vi "Periodic Tasks.vi"(8 "error in":errorcluster) -> ()   [LabVIEW 2017]
doc: "This VI runs in parallel to other tasks. It can contain as many user-defined periodic loops as you need. These can carry out PID or other sorts of timed response."
uses:
  <vilib>/Rock Robotics/WPI/DriverStation/WPI_DriverStationRobotMode2.ctl
  Robot Global Data.vi
  <vilib>/Rock Robotics/Network Tables/NT Write Boolean.vi
  Public/Documents/Cross The Road Electronics/Phoenix-LabVIEW/Motor Controller/Get/CTRE_Phoenix_MotorController_GetPulseWidthAll.vi
  <vilib>/Rock Robotics/Network Tables/NT Write Number.vi
  <vilib>/Rock Robotics/Network Tables/NT Read Boolean Array.vi
  <vilib>/Rock Robotics/Network Tables/NT Write Numeric Array.vi
  <vilib>/Utility/file.llb/Write Delimited Spreadsheet (DBL).vi
  <vilib>/Utility/file.llb/Read Delimited Spreadsheet (DBL).vi
  <vilib>/Rock Robotics/Network Tables/NT Read String.vi
  <vilib>/Rock Robotics/Network Tables/NT Write String.vi
  <vilib>/Rock Robotics/Network Tables/NT Read Numeric Array.vi
  <vilib>/Rock Robotics/Network Tables/NT Read Boolean.vi
  <vilib>/Rock Robotics/Network Tables/NT Read String Array.vi
  <vilib>/Rock Robotics/Network Tables/NT Write String Array.vi
panel:
  in  "Zero Gyro":bool
  in  "Enable Graphs":bool
  out "FL Drive":dbl(graph)
  out "FR Drive":dbl(graph)
  out "BL Drive 2":dbl(graph)
  out "BR Drive 2":dbl(graph)
  out "FL Spin 2":dbl(graph)
  out "BL Spin 3":dbl(graph)
  out "FR Spin 2":dbl(graph)
  out "BR Spin 3":dbl(graph)
  in  "Reset Lift at Start Config":bool
  in  "Disable DB Config Writing":bool
  in  "Save Zeros to File":bool
  in  "Read Zeros from File":bool
  in  "Zero Drive":bool
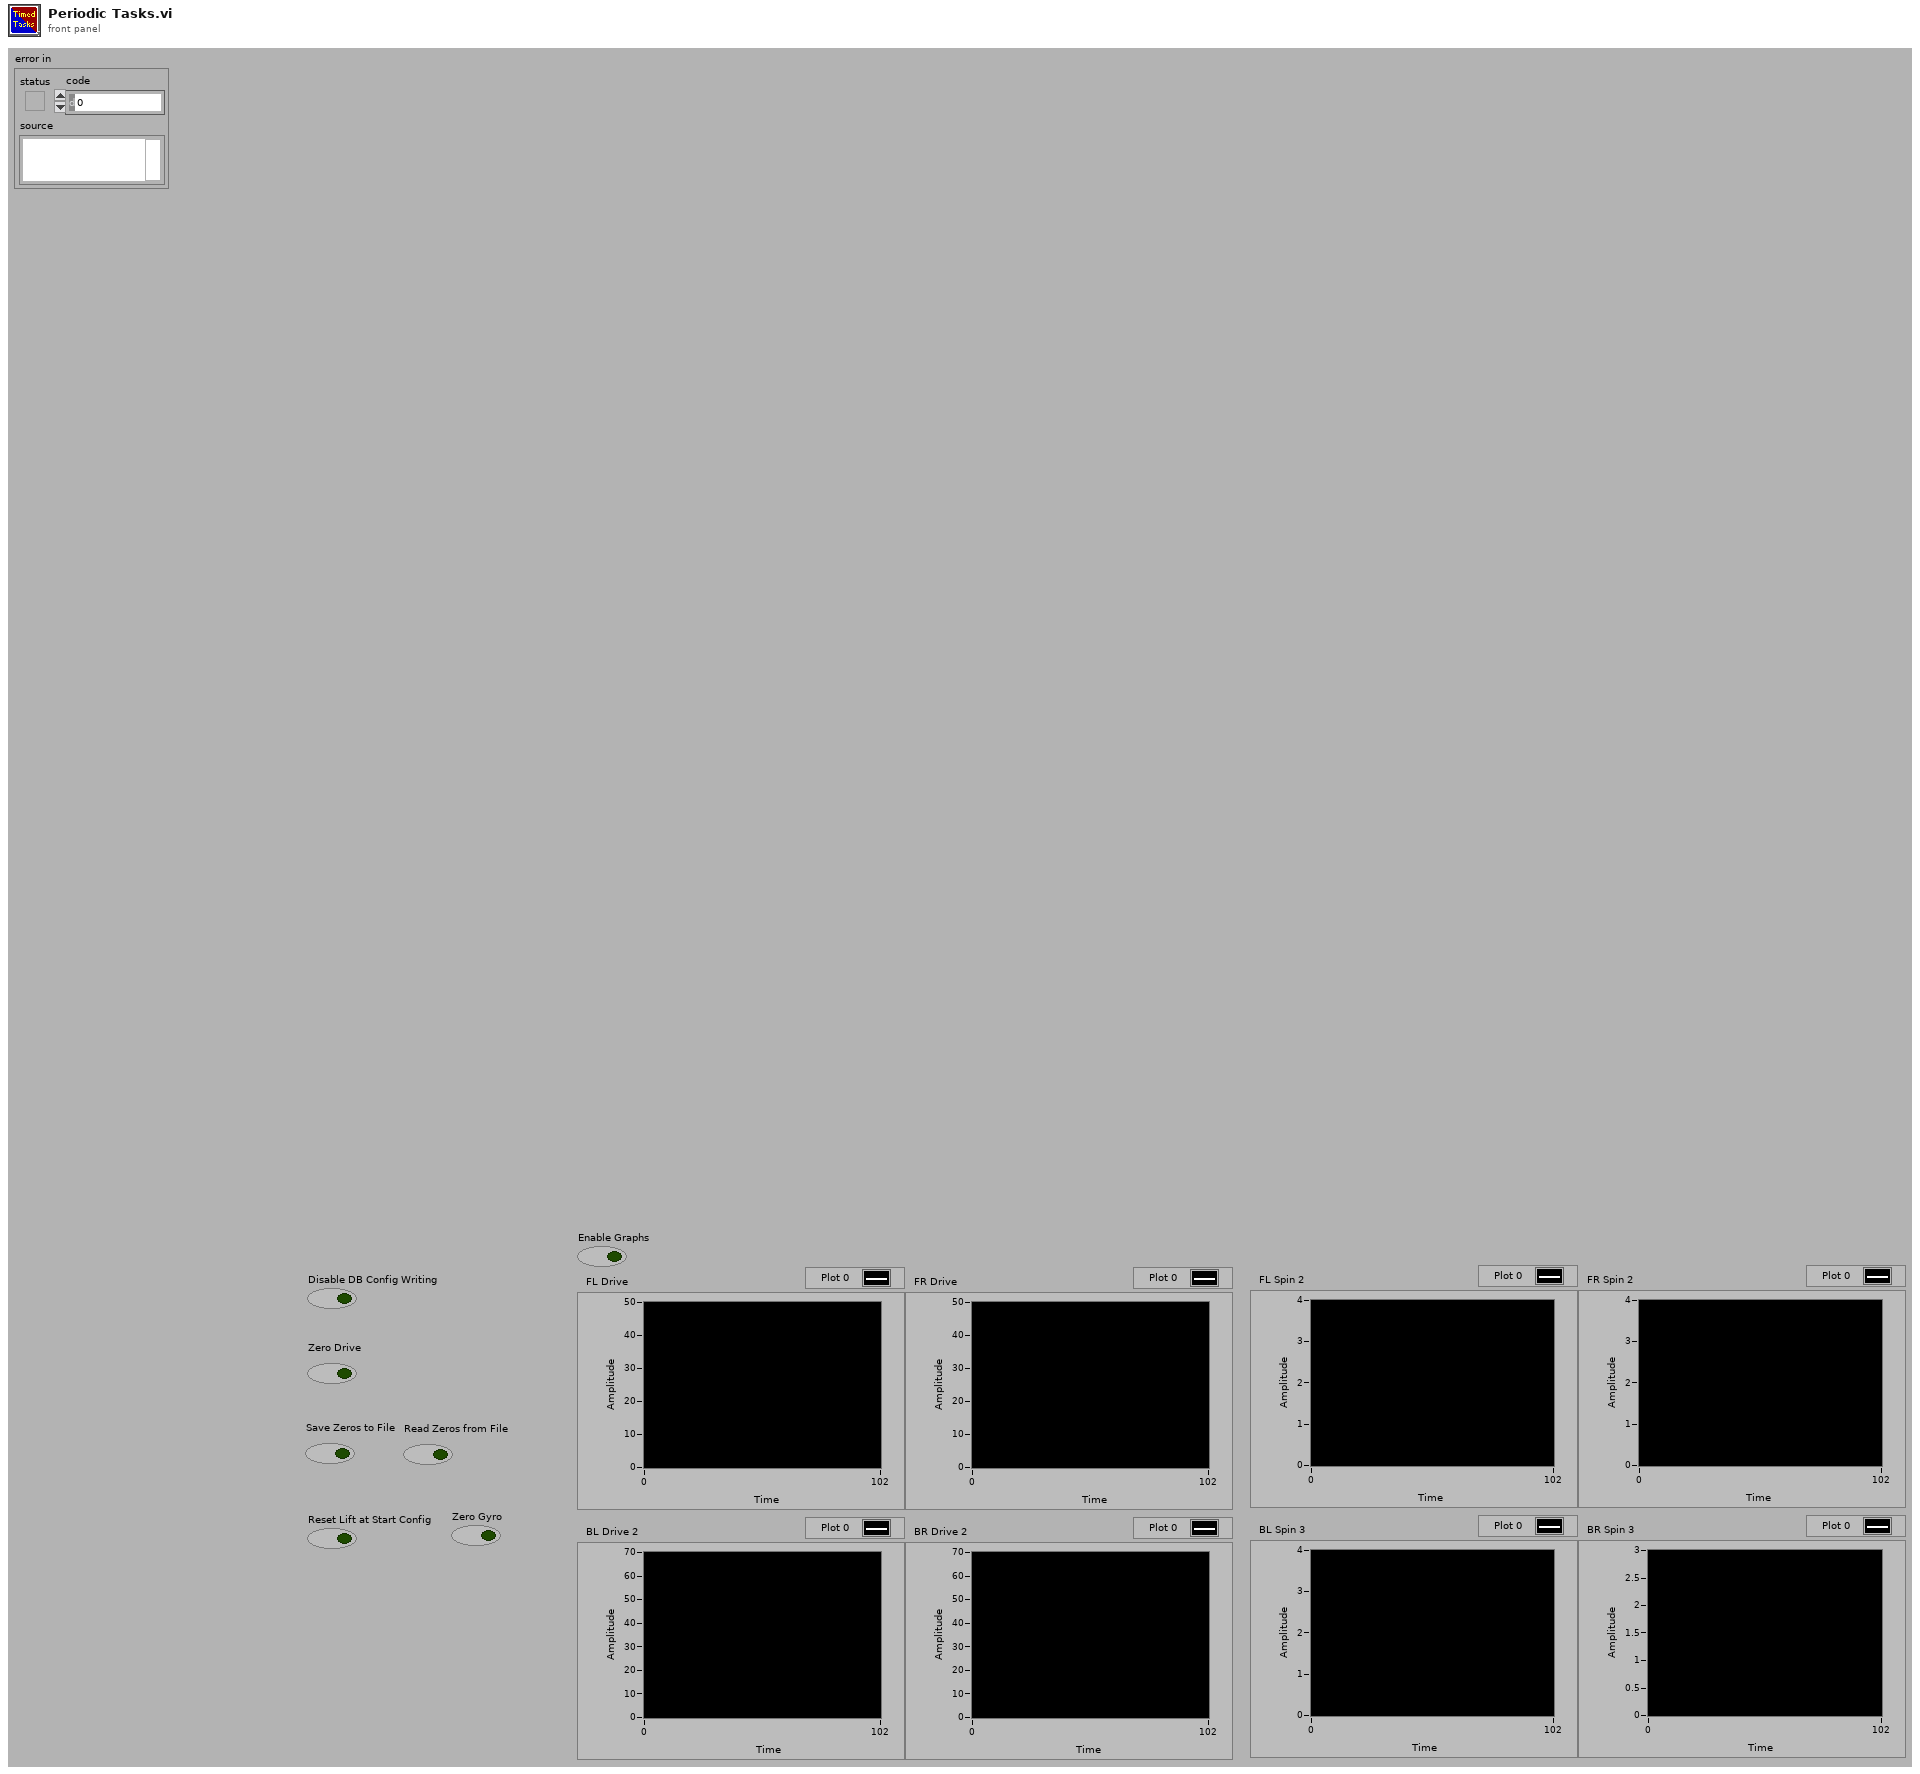
[diagram p1: front panel]
types:
  T1 = typedef "WPI_DriverStationRobotMode2.ctl" = enum16{"Autonomous Disabled", "Autonomous Enabled", "Teleop Disabled", "Teleop Enabled", "Disconnected", "Finish", "Test Disabled", "Test Enabled", "Emergency Stopped"}
  T2 = typedef "WPI_MotorControlDeviceRef.ctl" = cluster{"DeviceStatus":errorcluster, "Type":T3, "PWM":cluster{"PWM Channel":T4, "DeadBand":T5}, "CAN":cluster{"Device Number":u8, "SetOutput VI Ref":variant, "GetOutput VI Ref":variant, "Enable VI Ref":variant, "Disable VI Ref":variant, "Data":variant}, "Invert":bool, "DIO PWM":cluster{"PWM \"Enable\" Channel":T4, "DIOChannel":T6, "PWM Rate":dbl}}
  T3 = typedef "WPI_MotorControlType.ctl" = enum16{"PWM", "CAN", "DIO PWM"}
  T4 = typedef "FPGA_DIOPWMChannel.ctl" = enum8{"PWM 0", "PWM 1", "PWM 2", "PWM 3", "PWM 4", "PWM 5", "PWM 6", "PWM 7", "PWM 8", "PWM 9", "PWM MXP 0", "PWM MXP 1", "PWM MXP 2", "PWM MXP 3", "PWM MXP 4", "PWM MXP 5", "PWM MXP 6", "PWM MXP 7", "PWM MXP 8", "PWM MXP 9", "Invalid"}
  T5 = typedef "WPI_PWMDeadband.ctl" = cluster{"Name":string, "maxPositivePwm":i32, "minPositivePwm":i32, "centerPwm":i32, "maxNegativePwm":i32, "minNegativePwm":i32, "angularRange":u16}
  T6 = typedef "FPGA_DIOChannel.ctl" = enum8{"DIO 0", "DIO 1", "DIO 2", "DIO 3", "DIO 4", "DIO 5", "DIO 6", "DIO 7", "DIO 8", "DIO 9", "DIO MXP 0", "DIO MXP 1", "DIO MXP 2", "DIO MXP 3", "DIO MXP 4", "DIO MXP 5", "DIO MXP 6", "DIO MXP 7", "DIO MXP 8", "DIO MXP 9", "DIO MXP 10", "DIO MXP 11", "DIO MXP 12", "DIO MXP 13", "DIO MXP 14", "DIO MXP 15", "SPI Port CS1", "SPI Port CS2", "SPI Port CS3", "SPI Port MISO", "SPI Port MOSI", "Invalid"}
  T7 = typedef "WPI_SwitchDevRef.ctl" = cluster{"DevStatus":errorcluster, "DIO Channel":T6, "CntIndex":T8, "Normally Closed":bool}
  T8 = typedef "FPGA_CounterCtrSystemIndex.ctl" = enum8{"Ctr 0", "Ctr 1", "Ctr 2", "Ctr 3", "Ctr 4", "Ctr 5", "Ctr 6", "Ctr 7", "Invalid"}
  T9 = cluster{"Yaw":dbl, "Roll":dbl, "Pitch":dbl, "Heading":dbl, "Fused Heading":dbl}
  T10 = typedef "WPI_EncoderDevRef.ctl" = cluster{"DevStatus":errorcluster, "EncoderIndex":T11, "CounterIndex":T8, "DistancePerCount":dbl, "Decoding Type":T12}
  T11 = typedef "FPGA_EncoderIdx.ctl" = enum8{"Enc 0", "Enc 1", "Enc 2", "Enc 3", "Enc 4", "Enc 5", "Enc 6", "Enc 7", "Invalid"}
  T12 = typedef "WPI_EncoderType.ctl" = enum16{"1x", "2x", "4x"}
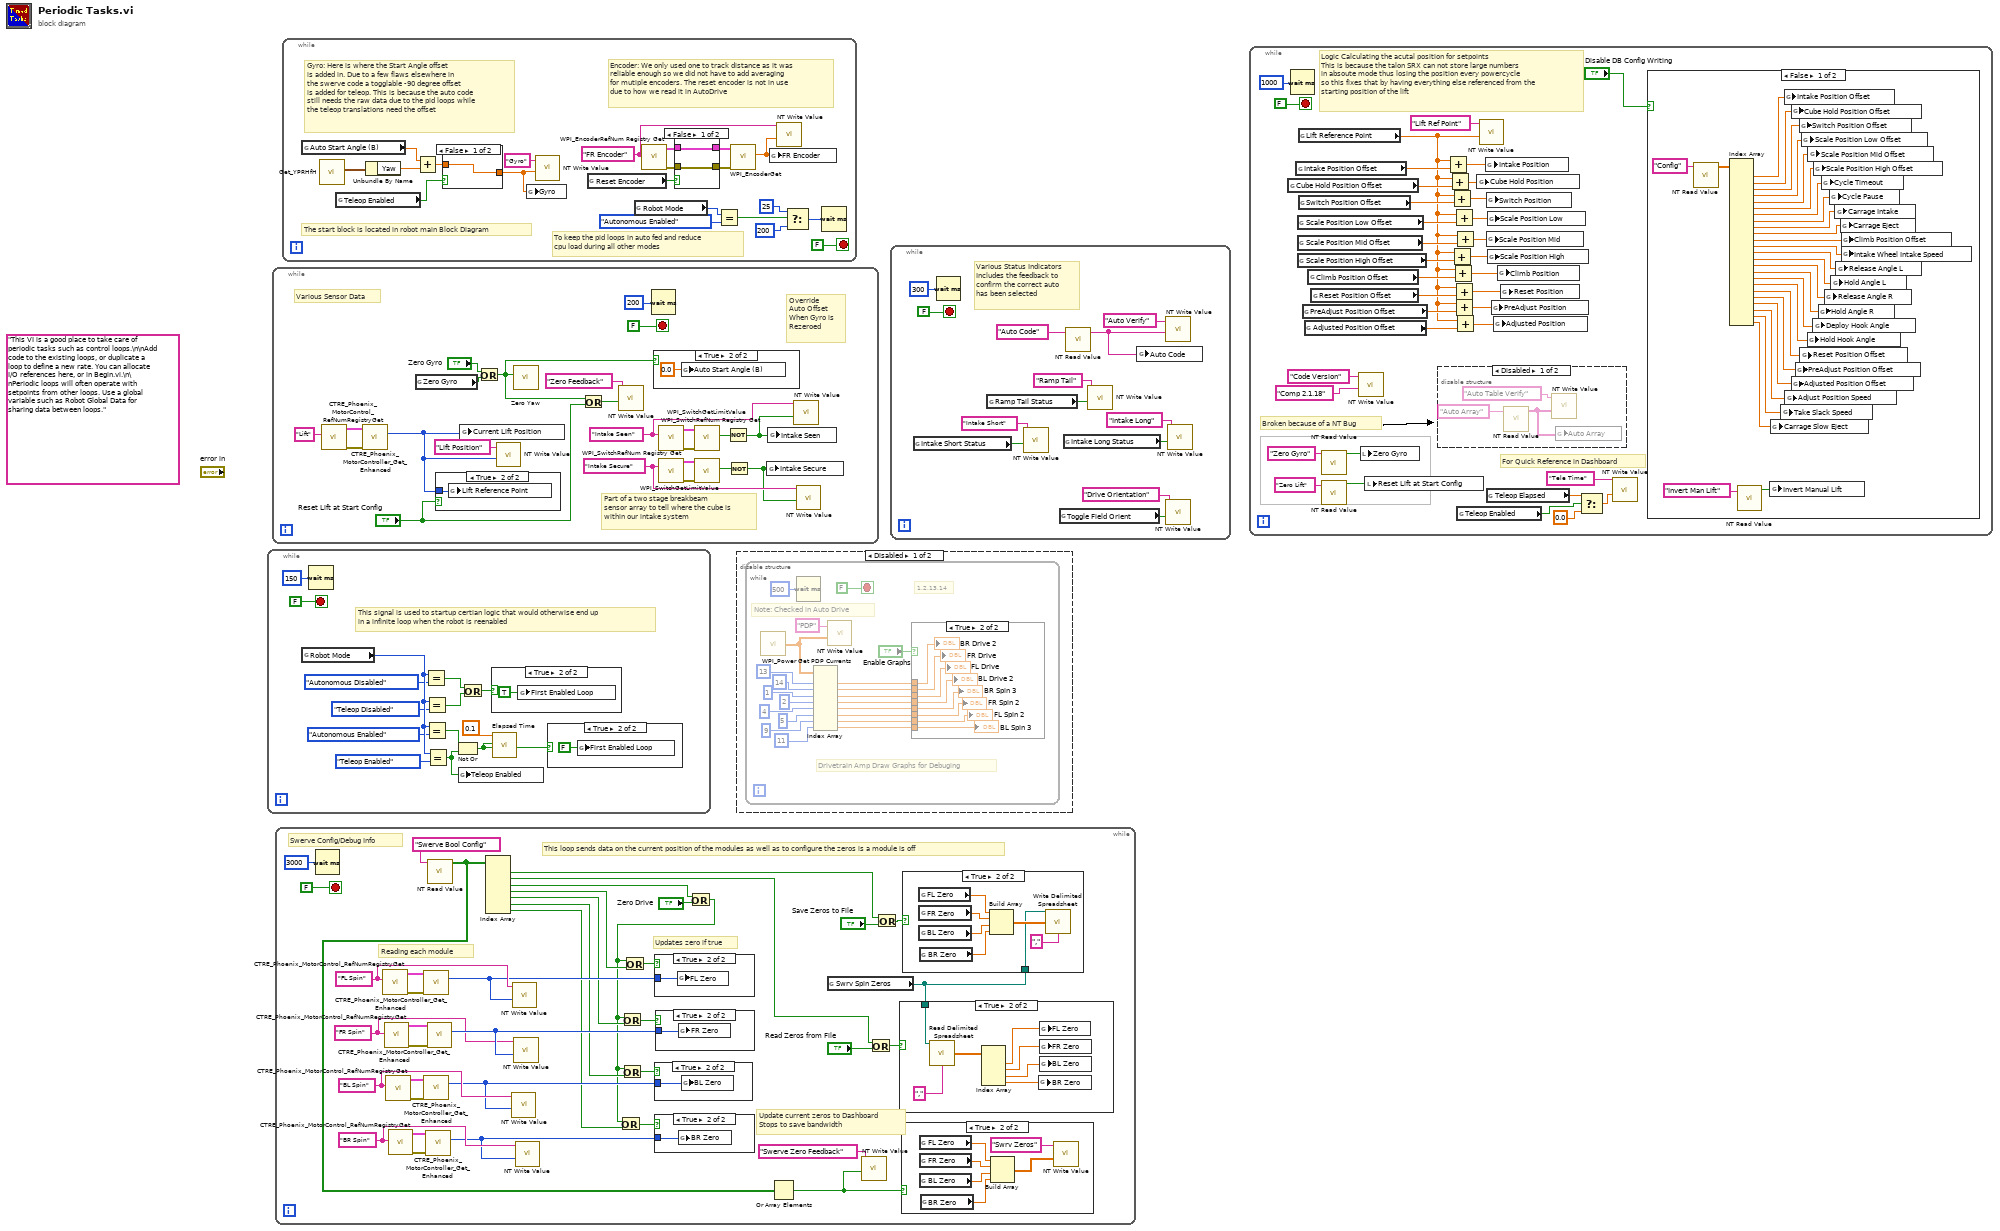
[diagram p0: block diagram]
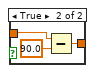
[diagram p2: hidden frame]
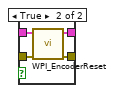
[diagram p3: hidden frame]
diagram:
  (unwired) "This VI is a good place to take care of periodic tasks such as control loops.\n\nAdd code to the existing loops, or duplicate a loop to define a new rate. You can allocate I/O references here, or in Begin.vi.\n\nPeriodic loops will often operate with setpoints from other loops. Use a global variable such as Robot Global Data for sharing data between loops."
  n1 = while {
    stop <- FALSE stop-if-true
    # "This signal is used to startup certian logic that would otherwise end up \nin a infinite loop when the robot is reenabled"
    n2 = global read "Robot Global Data.vi" "Robot Mode"() -> (w7:T1)
    n3 = Wait (ms)(milliseconds to wait=u32 150) -> ()  [unwired: 1 out]
    n4 = Equal?(x=w7, y=WPI_DriverStationRobotMode2."Autonomous Disabled") -> (x = y?=w8:bool)
    n5 = Equal?(x=w7, y=WPI_DriverStationRobotMode2."Teleop Disabled") -> (x = y?=w9:bool)
    n6 = Equal?(x=w7, y=WPI_DriverStationRobotMode2."Autonomous Enabled") -> (x = y?=w10:bool)
    n7 = Equal?(x=w7, y=WPI_DriverStationRobotMode2."Teleop Enabled") -> (x = y?=w1:bool)
    n8 = Not Or(1:w1, 2:w10) -> (0:w12:bool)
    n9 = global write "Robot Global Data.vi" "Teleop Enabled"(w1) -> ()
    n10 = Or(x=w8, y=w9) -> (x .or. y?=w11:bool)
    n11 = case shown="True" w11 {
      frame False {
      }
      frame True {
        n12 = global write "Robot Global Data.vi" "First Enabled Loop"(TRUE ("First Enabled Loop")) -> ()
      }
    }
    n13 = call "Elapsed Time"("Time Target (s)"=0.1, "Reset"=w12, "Auto Reset"=w12) -> ("Time has Elapsed"=w13:bool)  [unwired: 9 in, 7 out]
    n14 = case shown="True" w13 {
      frame False {
      }
      frame True {
        n15 = global write "Robot Global Data.vi" "First Enabled Loop"(FALSE ("First Enabled Loop")) -> ()
      }
    }
  }
  n16 = while {
    stop <- FALSE stop-if-true
    w32 = "Intake Secure" ("refnum name")
    w31 = "Intake Seen" ("refnum name")
    # "Part of a two stage breakbeam\nsensor array to tell where the cube is\nwithin our intake system"
    # "Override\nAuto Offset\nWhen Gyro is\nRezeroed"
    # "Various Sensor Data"
    n17 = call "CTRE_Phoenix_MotorControl_RefNumRegistryGet.vi"("refnum name"="Lift") -> ("error out"=w28:errorcluster, "PhoenixMotorControlDevRef"=w29:T2)  [unwired: 9 in]
    n18 = call-poly "CTRE_Phoenix_MotorController_Get_Enhanced.vi"("PhoenixMotorControlDevRef"=w29, "error in"=w28) -> ("Pulse Width Position"=w23:i32)  [unwired: 8 in, 5 out]
    n19 = global read "Robot Global Data.vi" "Zero Gyro"() -> (w20:bool)
    n20 = case shown="True" "Reset Lift at Start Config" {
      tunnel: w23 -> [_ w42]
      frame False {
      }
      frame True {
        n21 = global write "Robot Global Data.vi" "Lift Reference Point"(w42) -> ()
      }
    }
    n22 = global write "Robot Global Data.vi" "Current Lift Position"(w23) -> ()
    n23 = Or(x="Zero Gyro", y=w20) -> (x .or. y?=w18:bool)
    n24 = call-poly <vilib>:"NT Write Value.vi"("Numeric"=w23, "Name"="Lift Position") -> ()  [unwired: 9 in, 1 out]
    n25 = call <vilib>:"Zero Yaw.vi"("Zero"=w18) -> ()  [unwired: 11 in]
    n26 = Or(x=w18, y="Reset Lift at Start Config") -> (x .or. y?=w21:bool)
    n27 = call-poly <vilib>:"NT Write Value.vi"("Boolean"=w21, "Name"="Zero Feedback") -> ()  [unwired: 9 in, 1 out]
    n28 = Wait (ms)(milliseconds to wait=u32 200) -> ()  [unwired: 1 out]
    n29 = case shown="True" w18 {
      frame False {
      }
      frame True {
        n30 = global write "Robot Global Data.vi" "Auto Start Angle (B)"(0.0 ("Auto Start Angle (B)")) -> ()
      }
    }
    n31 = call <vilib>:"WPI_SwitchRefNum Registry Get.vi"("refnum name"=w31) -> ("error out"=w37:errorcluster, "SwitchDevRef"=w36:T7)  [unwired: 9 in]
    n32 = call <vilib>:"WPI_SwitchRefNum Registry Get.vi"("refnum name"=w32) -> ("error out"=w35:errorcluster, "SwitchDevRef"=w34:T7)  [unwired: 9 in]
    n33 = call <vilib>:"WPI_SwitchGetLimitValue.vi"("error in (no error)"=w37, "SwitchDevRef"=w36) -> ("Switch Pressed"=w38:bool)  [unwired: 7 in, 2 out]
    n34 = call <vilib>:"WPI_SwitchGetLimitValue.vi"("error in (no error)"=w35, "SwitchDevRef"=w34) -> ("Switch Pressed"=w33:bool)  [unwired: 7 in, 2 out]
    n35 = Not(x=w38) -> (.not. x?=w26:bool)
    n36 = Not(x=w33) -> (.not. x?=w25:bool)
    n37 = global write "Robot Global Data.vi" "Intake Secure"(w25) -> ()
    n38 = global write "Robot Global Data.vi" "Intake Seen"(w26) -> ()
    n39 = call-poly <vilib>:"NT Write Value.vi"("Boolean"=w26, "Name"=w31) -> ()  [unwired: 9 in, 1 out]
    n40 = call-poly <vilib>:"NT Write Value.vi"("Boolean"=w25, "Name"=w32) -> ()  [unwired: 9 in, 1 out]
  }
  n41 = while {
    stop <- FALSE stop-if-true
    w65 = "BR Spin" ("refnum name")
    w67 = "BL Spin" ("refnum name")
    w68 = "FR Spin" ("refnum name")
    w71 = "FL Spin" ("refnum name")
    # "Reading each module"
    # "Updates zero if true"
    # "This loop sends data on the current position of the modules as well as to configure the zeros is a module is off"
    # "Update current zeros to Dashboard\nStops to save bandwidth"
    # "Swerve Config/Debug Info"
    n42 = Wait (ms)(milliseconds to wait=u32 3000) -> ()  [unwired: 1 out]
    n43 = call "CTRE_Phoenix_MotorControl_RefNumRegistryGet.vi"("refnum name"=w71) -> ("error out"=w73:errorcluster, "PhoenixMotorControlDevRef"=w72:T2)  [unwired: 9 in]
    n44 = call "CTRE_Phoenix_MotorControl_RefNumRegistryGet.vi"("refnum name"=w68) -> ("error out"=w75:errorcluster, "PhoenixMotorControlDevRef"=w74:T2)  [unwired: 9 in]
    n45 = call "CTRE_Phoenix_MotorControl_RefNumRegistryGet.vi"("refnum name"=w67) -> ("error out"=w77:errorcluster, "PhoenixMotorControlDevRef"=w76:T2)  [unwired: 9 in]
    n46 = call "CTRE_Phoenix_MotorControl_RefNumRegistryGet.vi"("refnum name"=w65) -> ("error out"=w79:errorcluster, "PhoenixMotorControlDevRef"=w78:T2)  [unwired: 9 in]
    n47 = call-poly "CTRE_Phoenix_MotorController_Get_Enhanced.vi"("PhoenixMotorControlDevRef"=w72, "error in"=w73) -> ("Pulse Width Position"=w70:i32)  [unwired: 8 in, 5 out]
    n48 = call-poly "CTRE_Phoenix_MotorController_Get_Enhanced.vi"("PhoenixMotorControlDevRef"=w76, "error in"=w77) -> ("Pulse Width Position"=w66:i32)  [unwired: 8 in, 5 out]
    n49 = call-poly "CTRE_Phoenix_MotorController_Get_Enhanced.vi"("PhoenixMotorControlDevRef"=w78, "error in"=w79) -> ("Pulse Width Position"=w64:i32)  [unwired: 8 in, 5 out]
    n50 = call-poly "CTRE_Phoenix_MotorController_Get_Enhanced.vi"("PhoenixMotorControlDevRef"=w74, "error in"=w75) -> ("Pulse Width Position"=w69:i32)  [unwired: 8 in, 5 out]
    n51 = call-poly <vilib>:"NT Read Value.vi"("Name"="Swerve Bool Config") -> ("Boolean Array"=w45:bool[])  [unwired: 9 in, 1 out]
    n52 = Index Array(array=w45) -> (element #1=w55:bool, element #2=w56:bool, element #3=w57:bool, element #4=w54:bool, element #5=w53:bool, element #6=w52:bool, element #7=w51:bool)  [unwired: 7 in]
    n53 = call-poly <vilib>:"NT Write Value.vi"("Numeric"=w66, "Name"=w67) -> ()  [unwired: 9 in, 1 out]
    n54 = call-poly <vilib>:"NT Write Value.vi"("Numeric"=w70, "Name"=w71) -> ()  [unwired: 9 in, 1 out]
    n55 = call-poly <vilib>:"NT Write Value.vi"("Numeric"=w69, "Name"=w68) -> ()  [unwired: 9 in, 1 out]
    n56 = call-poly <vilib>:"NT Write Value.vi"("Numeric"=w64, "Name"=w65) -> ()  [unwired: 9 in, 1 out]
    n57 = Or(x=w57, y="Zero Drive") -> (x .or. y?=w46:bool)
    n58 = Or(x=w46, y=w51) -> (x .or. y?=w47:bool)
    n59 = Or(x=w46, y=w53) -> (x .or. y?=w49:bool)
    n60 = Or(x=w46, y=w52) -> (x .or. y?=w48:bool)
    n61 = Or(x=w46, y=w54) -> (x .or. y?=w50:bool)
    n62 = case shown="True" w50 {
      tunnel: w70 -> [_ w92]
      frame False {
      }
      frame True {
        n63 = global write "Robot Global Data.vi" "FL Zero"(w92) -> ()
      }
    }
    n64 = case shown="True" w48 {
      tunnel: w66 -> [_ w90]
      frame False {
      }
      frame True {
        n65 = global write "Robot Global Data.vi" "BL Zero"(w90) -> ()
      }
    }
    n66 = case shown="True" w47 {
      tunnel: w64 -> [_ w89]
      frame False {
      }
      frame True {
        n67 = global write "Robot Global Data.vi" "BR Zero"(w89) -> ()
      }
    }
    n68 = case shown="True" w49 {
      tunnel: w69 -> [_ w91]
      frame False {
      }
      frame True {
        n69 = global write "Robot Global Data.vi" "FR Zero"(w91) -> ()
      }
    }
    n70 = Or Array Elements(Boolean array=w45) -> (logical OR=w43:bool)
    n71 = global read "Robot Global Data.vi" "Swrv Spin Zeros"() -> (w80:path)
    n72 = call-poly <vilib>:"NT Write Value.vi"("Boolean"=w43, "Name"="Swerve Zero Feedback") -> ()  [unwired: 9 in, 1 out]
    n73 = Or(x=w56, y="Read Zeros from File") -> (x .or. y?=w61:bool)
    n74 = Or(x=w55, y="Save Zeros to File") -> (x .or. y?=w60:bool)
    n75 = case shown="True" w61 {
      tunnel: w80 -> [_ w99]
      frame False {
      }
      frame True {
        n76 = call-poly <vilib>:"Read Delimited Spreadsheet.vi"("file path (dialog if empty)"=w99, "delimiter (\\t)"="," ("delimiter (\\t)")) -> ("first row"=w98:dbl[])  [unwired: 8 in, 5 out]
        n77 = Index Array(array=w98) -> (element #1=w93:dbl, element #2=w94:dbl, element #3=w95:dbl, element #4=w96:dbl)  [unwired: 4 in]
        n78 = global write "Robot Global Data.vi" "BR Zero"(w96) -> ()
        n79 = global write "Robot Global Data.vi" "FL Zero"(w93) -> ()
        n80 = global write "Robot Global Data.vi" "FR Zero"(w94) -> ()
        n81 = global write "Robot Global Data.vi" "BL Zero"(w95) -> ()
      }
    }
    n82 = case shown="True" w43 {
      frame False {
      }
      frame True {
        n83 = global read "Robot Global Data.vi" "FL Zero"() -> (w85:dbl)
        n84 = global read "Robot Global Data.vi" "FR Zero"() -> (w86:dbl)
        n85 = global read "Robot Global Data.vi" "BL Zero"() -> (w87:dbl)
        n86 = global read "Robot Global Data.vi" "BR Zero"() -> (w84:dbl)
        n87 = Build Array(w85, w86, w87, w84) -> (w83:dbl[])
        n88 = call-poly <vilib>:"NT Write Value.vi"("Numeric Array"=w83, "Name"="Swrv Zeros") -> ()  [unwired: 9 in, 1 out]
      }
    }
    n89 = case shown="True" w60 {
      tunnel: w80 -> [_ w101]
      frame False {
      }
      frame True {
        n90 = global read "Robot Global Data.vi" "FL Zero"() -> (w104:dbl)
        n91 = global read "Robot Global Data.vi" "FR Zero"() -> (w105:dbl)
        n92 = global read "Robot Global Data.vi" "BL Zero"() -> (w106:dbl)
        n93 = global read "Robot Global Data.vi" "BR Zero"() -> (w103:dbl)
        n94 = Build Array(w104, w105, w106, w103) -> (w102:dbl[])
        n95 = call-poly <vilib>:"Write Delimited Spreadsheet.vi"("file path (dialog if empty)"=w101, "1D data"=w102, "delimiter (\\t)"="," ("delimiter (\\t)")) -> ()  [unwired: 11 in, 2 out]
      }
    }
  }
  n96 = while {
    stop <- FALSE stop-if-true
    w114 = "FR Encoder" ("refnum name")
    # "To keep the pid loops in auto fed and reduce\ncpu load during all other modes"
    # "Encoder: We only used one to track distance as it was\nreliable enough so we did not have to add averaging\nfor mutiple encoders. The reset encoder is not in use\ndue to how we read it in AutoDrive"
    # "The start block is located in robot main Block Diagram"
    # "Gyro: Here is where the Start Angle offset\nis added in. Due to a few flaws elsewhere in\nthe swerve code a togglable -90 degree offset\nis added for teleop. This is because the auto code\nstill needs the raw data due to the pid loops while\nthe teleop translations need the offset"
    n97 = global read "Robot Global Data.vi" "Auto Start Angle (B)"() -> (w113:dbl)
    n98 = call <vilib>:"Get_YPRHfH.vi"() -> ("YRPHfH"=w109:T9)  [unwired: 11 in]
    n99 = global read "Robot Global Data.vi" "Teleop Enabled"() -> (w107:bool)
    n100 = Unbundle By Name(w109) -> ("Yaw"=w112:dbl)
    n101 = Add(x=w113, y=w112) -> (x+y=w111:dbl)
    n102 = case shown="False" w107 {
      tunnel: [w128 w131] -> w110
      tunnel: w111 -> [w128 w130]
      frame False {
      }
      frame True {
        n103 = Subtract(x=w130, y=90.0) -> (x-y=w131:dbl)
      }
    }
    n104 = global write "Robot Global Data.vi" "Gyro"(w110) -> ()
    n105 = call-poly <vilib>:"NT Write Value.vi"("Numeric"=w110, "Name"="Gyro") -> ()  [unwired: 9 in, 1 out]
    n106 = global read "Robot Global Data.vi" "Reset Encoder"() -> (w119:bool)
    n107 = global read "Robot Global Data.vi" "Robot Mode"() -> (w123:T1)
    n108 = call <vilib>:"WPI_EncoderRefNum Registry Get.vi"("refnum name"=w114) -> ("error out"=w115:errorcluster, "EncoderDevRef"=w116:T10)  [unwired: 9 in]
    n109 = case shown="False" w119 {
      tunnel: w115 -> [w132 w137]
      tunnel: w116 -> [w133 w136]
      tunnel: [w133 w135] -> w117
      tunnel: [w132 w134] -> w118
      frame False {
      }
      frame True {
        n110 = call <vilib>:"WPI_EncoderReset.vi"("error in (no error)"=w137, "EncoderDevRef"=w136) -> ("error out"=w134:errorcluster, "EncoderDevRef"=w135:T10)  [unwired: 8 in]
      }
    }
    n111 = Equal?(x=w123, y=WPI_DriverStationRobotMode2."Autonomous Enabled") -> (x = y?=w121:bool)
    n112 = call <vilib>:"WPI_EncoderGet.vi"("error in (no error)"=w118, "EncoderDevRef"=w117) -> ("Distance"=w120:dbl)  [unwired: 4 in, 5 out]
    n113 = global write "Robot Global Data.vi" "FR Encoder"(w120) -> ()
    n114 = call-poly <vilib>:"NT Write Value.vi"("Numeric"=w120, "Name"=w114) -> ()  [unwired: 9 in, 1 out]
    n115 = Select(t=u32 25, s=w121, f=u32 200 ("milliseconds to wait")) -> (s? t:f=w126:u32)
    n116 = Wait (ms)(milliseconds to wait=w126) -> ()  [unwired: 1 out]
  }
  n117 = disable-structure shown="Disabled" {
    frame Disabled {
      n118 = while {
        stop <- FALSE stop-if-true
        # "Drivetrain Amp Draw Graphs for Debuging"
        # "Note: Checked in Auto Drive"
        # "1,2,13,14"
        n119 = call <vilib>:"WPI_Power Get PDP Currents.vi"() -> ("all currents (A)"=w158:dbl[])  [unwired: 13 in, 2 out]
        n120 = Wait (ms)(milliseconds to wait=u32 500) -> ()  [unwired: 1 out]
        n121 = Index Array(array=w158, index #1=13 ("index"), index #2=14 ("index"), index #3=1 ("index"), index #4=2 ("index"), index #5=4 ("index"), index #6=5 ("index"), index #7=9 ("index"), index #8=11 ("index")) -> (element #1=w149:dbl, element #2=w153:dbl, element #3=w156:dbl, element #4=w152:dbl, element #5=w150:dbl, element #6=w154:dbl, element #7=w155:dbl, element #8=w151:dbl)
        n122 = call-poly <vilib>:"NT Write Value.vi"("Numeric Array"=w158, "Name"="PDP") -> ()  [unwired: 9 in, 1 out]
        n123 = case shown="True" "Enable Graphs" {
          tunnel: w149 -> [_ w166]
          tunnel: w150 -> [_ w165]
          tunnel: w151 -> [_ w164]
          tunnel: w152 -> [_ w163]
          tunnel: w153 -> [_ w162]
          tunnel: w154 -> [_ w161]
          tunnel: w155 -> [_ w160]
          tunnel: w156 -> [_ w159]
          frame False {
          }
          frame True {
            "FL Drive" <- w159
            "FR Drive" <- w162
            "BL Drive 2" <- w163
            "BR Drive 2" <- w166
            "FL Spin 2" <- w160
            "BL Spin 3" <- w164
            "FR Spin 2" <- w161
            "BR Spin 3" <- w165
          }
        }
      }
    }
    frame Enabled {
    }
  }
  n124 = while {
    stop <- FALSE stop-if-true
    # "Various Status Indicators\nIncludes the feedback to\nconfirm the correct auto\nhas been selected"
    n125 = global read "Robot Global Data.vi" "Intake Short Status"() -> (w171:bool)
    n126 = Wait (ms)(milliseconds to wait=u32 300) -> ()  [unwired: 1 out]
    n127 = global read "Robot Global Data.vi" "Ramp Tail Status"() -> (w173:bool)
    n128 = call-poly <vilib>:"NT Write Value.vi"("Boolean"=w171, "Name"="Intake Short") -> ()  [unwired: 9 in, 1 out]
    n129 = global read "Robot Global Data.vi" "Toggle Field Orient"() -> (w175:bool)
    n130 = global read "Robot Global Data.vi" "Intake Long Status"() -> (w172:bool)
    n131 = call-poly <vilib>:"NT Read Value.vi"("Name"="Auto Code") -> ("String"=w167:string)  [unwired: 9 in, 1 out]
    n132 = call-poly <vilib>:"NT Write Value.vi"("Boolean"=w173, "Name"="Ramp Tail") -> ()  [unwired: 9 in, 1 out]
    n133 = global write "Robot Global Data.vi" "Auto Code"(w167) -> ()
    n134 = call-poly <vilib>:"NT Write Value.vi"("String"=w167, "Name"="Auto Verify") -> ()  [unwired: 9 in, 1 out]
    n135 = call-poly <vilib>:"NT Write Value.vi"("Boolean"=w175, "Name"="Drive Orientation") -> ()  [unwired: 9 in, 1 out]
    n136 = call-poly <vilib>:"NT Write Value.vi"("Boolean"=w172, "Name"="Intake Long") -> ()  [unwired: 9 in, 1 out]
  }
  n137 = while {
    stop <- FALSE stop-if-true
    # "Logic Calculating the acutal position for setpoints\nThis is because the talon SRX can not store large numbers\nin absoute mode thus losing the position every powercycle\nso this fixes that by having everything else referenced from the\nstarting position of the lift"
    # "For Quick Reference in Dashboard"
    # "Broken because of a NT Bug"
    n138 = global read "Robot Global Data.vi" "Cube Hold Position Offset"() -> (w204:dbl)
    n139 = Wait (ms)(milliseconds to wait=u32 1000) -> ()  [unwired: 1 out]
    n140 = global read "Robot Global Data.vi" "Intake Position Offset"() -> (w200:dbl)
    n141 = global read "Robot Global Data.vi" "Scale Position Low Offset"() -> (w206:dbl)
    n142 = global read "Robot Global Data.vi" "Scale Position Mid Offset"() -> (w207:dbl)
    n143 = global read "Robot Global Data.vi" "Scale Position High Offset"() -> (w208:dbl)
    n144 = global read "Robot Global Data.vi" "Lift Reference Point"() -> (w185:dbl)
    n145 = global read "Robot Global Data.vi" "Switch Position Offset"() -> (w205:dbl)
    n146 = global read "Robot Global Data.vi" "PreAdjust Position Offset"() -> (w188:dbl)
    n147 = global read "Robot Global Data.vi" "Adjusted Position Offset"() -> (w186:dbl)
    n148 = global read "Robot Global Data.vi" "Climb Position Offset"() -> (w202:dbl)
    n149 = global read "Robot Global Data.vi" "Reset Position Offset"() -> (w197:dbl)
    n150 = call-poly <vilib>:"NT Read Value.vi"("Name"="Zero Gyro") -> ("Boolean"=w191:bool)  [unwired: 9 in, 1 out]
    n151 = call-poly <vilib>:"NT Read Value.vi"("Name"="Zero Lift") -> ("Boolean"=w190:bool)  [unwired: 9 in, 1 out]
    n152 = call-poly <vilib>:"NT Write Value.vi"("String"="Comp 2.1.18", "Name"="Code Version") -> ()  [unwired: 9 in, 1 out]
    n153 = local write "Zero Gyro"(w191) -> ()
    n154 = local write "Reset Lift at Start Config"(w190) -> ()
    n155 = disable-structure shown="Disabled" {
      frame Disabled {
        n156 = call-poly <vilib>:"NT Read Value.vi"("Name"="Auto Array") -> ("String Array"=w216:string[])  [unwired: 9 in, 1 out]
        n157 = call-poly <vilib>:"NT Write Value.vi"("String Array"=w216, "Name"="Auto Table Verify") -> ()  [unwired: 9 in, 1 out]
        n158 = global write "Robot Global Data.vi" "Auto Array"(w216) -> ()
      }
      frame Enabled {
      }
    }
    n159 = Add(x=w185, y=w200) -> (x+y=w201:dbl)
    n160 = Add(x=w185, y=w204) -> (x+y=w213:dbl)
    n161 = Add(x=w185, y=w205) -> (x+y=w212:dbl)
    n162 = Add(x=w185, y=w208) -> (x+y=w209:dbl)
    n163 = Add(x=w185, y=w202) -> (x+y=w203:dbl)
    n164 = Add(x=w185, y=w206) -> (x+y=w211:dbl)
    n165 = Add(x=w185, y=w197) -> (x+y=w198:dbl)
    n166 = Add(x=w185, y=w188) -> (x+y=w189:dbl)
    n167 = Add(x=w185, y=w207) -> (x+y=w210:dbl)
    n168 = Add(x=w185, y=w186) -> (x+y=w187:dbl)
    n169 = global read "Robot Global Data.vi" "Teleop Enabled"() -> (w181:bool)
    n170 = global write "Robot Global Data.vi" "Cube Hold Position"(w213) -> ()
    n171 = call-poly <vilib>:"NT Write Value.vi"("Numeric"=w185, "Name"="Lift Ref Point") -> ()  [unwired: 9 in, 1 out]
    n172 = global write "Robot Global Data.vi" "Intake Position"(w201) -> ()
    n173 = global write "Robot Global Data.vi" "Switch Position"(w212) -> ()
    n174 = global write "Robot Global Data.vi" "Scale Position Mid"(w210) -> ()
    n175 = global read "Robot Global Data.vi" "Teleop Elapsed"() -> (w182:dbl)
    n176 = global write "Robot Global Data.vi" "Scale Position Low"(w211) -> ()
    n177 = global write "Robot Global Data.vi" "Scale Position High"(w209) -> ()
    n178 = global write "Robot Global Data.vi" "PreAdjust Position"(w189) -> ()
    n179 = global write "Robot Global Data.vi" "Adjusted Position"(w187) -> ()
    n180 = global write "Robot Global Data.vi" "Climb Position"(w203) -> ()
    n181 = global write "Robot Global Data.vi" "Reset Position"(w198) -> ()
    n182 = Select(t=w182, s=w181, f=0.0) -> (s? t:f=w183:dbl)
    n183 = call-poly <vilib>:"NT Write Value.vi"("Numeric"=w183, "Name"="Tele Time") -> ()  [unwired: 9 in, 1 out]
    n184 = case shown="False" "Disable DB Config Writing" {
      frame False {
        n185 = call-poly <vilib>:"NT Read Value.vi"("Name"="Config") -> ("Numeric Array"=w245:dbl[])  [unwired: 9 in, 1 out]
        n186 = Index Array(array=w245) -> (element #1=w244:dbl, element #2=w243:dbl, element #3=w242:dbl, element #4=w241:dbl, element #5=w240:dbl, element #6=w239:dbl, element #7=w238:dbl, element #8=w237:dbl, element #9=w236:dbl, element #10=w235:dbl, element #11=w234:dbl, element #12=w233:dbl, element #13=w232:dbl, element #14=w231:dbl, element #15=w230:dbl, element #16=w229:dbl, element #17=w228:dbl, element #18=w227:dbl, element #19=w226:dbl, element #20=w223:dbl, element #21=w222:dbl, element #22=w221:dbl, element #23=w220:dbl, element #24=w219:dbl)  [unwired: 24 in]
        n187 = call-poly <vilib>:"NT Read Value.vi"("Name"="Invert Man Lift") -> ("Boolean"=w225:bool)  [unwired: 9 in, 1 out]
        n188 = global write "Robot Global Data.vi" "Invert Manual Lift"(w225) -> ()
        n189 = global write "Robot Global Data.vi" "Carrage Slow Eject"(w219) -> ()
        n190 = global write "Robot Global Data.vi" "Take Slack Speed"(w220) -> ()
        n191 = global write "Robot Global Data.vi" "Intake Position Offset"(w244) -> ()
        n192 = global write "Robot Global Data.vi" "Adjust Position Speed"(w221) -> ()
        n193 = global write "Robot Global Data.vi" "Cube Hold Position Offset"(w243) -> ()
        n194 = global write "Robot Global Data.vi" "Adjusted Position Offset"(w222) -> ()
        n195 = global write "Robot Global Data.vi" "PreAdjust Position Offset"(w223) -> ()
        n196 = global write "Robot Global Data.vi" "Switch Position Offset"(w242) -> ()
        n197 = global write "Robot Global Data.vi" "Reset Position Offset"(w226) -> ()
        n198 = global write "Robot Global Data.vi" "Scale Position Low Offset"(w241) -> ()
        n199 = global write "Robot Global Data.vi" "Hold Hook Angle"(w227) -> ()
        n200 = global write "Robot Global Data.vi" "Scale Position Mid Offset"(w240) -> ()
        n201 = global write "Robot Global Data.vi" "Deploy Hook Angle"(w228) -> ()
        n202 = global write "Robot Global Data.vi" "Scale Position High Offset"(w239) -> ()
        n203 = global write "Robot Global Data.vi" "Hold Angle R"(w229) -> ()
        n204 = global write "Robot Global Data.vi" "Cycle Timeout"(w238) -> ()
        n205 = global write "Robot Global Data.vi" "Release Angle R"(w230) -> ()
        n206 = global write "Robot Global Data.vi" "Cycle Pause"(w237) -> ()
        n207 = global write "Robot Global Data.vi" "Hold Angle L"(w231) -> ()
        n208 = global write "Robot Global Data.vi" "Carrage Intake"(w236) -> ()
        n209 = global write "Robot Global Data.vi" "Release Angle L"(w232) -> ()
        n210 = global write "Robot Global Data.vi" "Carrage Eject"(w235) -> ()
        n211 = global write "Robot Global Data.vi" "Climb Position Offset"(w234) -> ()
        n212 = global write "Robot Global Data.vi" "Intake Wheel Intake Speed"(w233) -> ()
      }
      frame True {
      }
    }
  }
